vi "Configure Marker Search.vi"(7 "Marker Search (Max Peak)":T1, 8 "error in (no error)":errorcluster, 10 "Marker Number (1)":u32=1 min=1, 11 "SA-FSW in":refnum<class "SA-FSW.lvclass">) -> (0 "error out":errorcluster, 3 "SA-FSW out":refnum<class "SA-FSW.lvclass">)   [LabVIEW 2020, in "SA-FSW.lvclass"]
uses:
  SA-FSW.lvclass
  C:/Sandbox/RF Bench/Source Code/WiSpry Test Framework/Instruments/Instrument.lvclass
  Controls/Marker Search.ctl
  Instrument.lvclass/Instrument.ctl
  Instrument.lvclass
  Spectrum Analyzer.lvclass
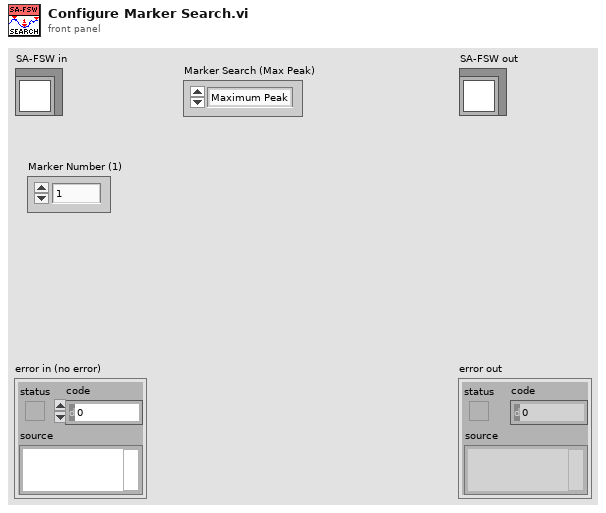
[diagram p1: front panel]
types:
  T1 = typedef "Spectrum Analyzer.lvclass/Marker Search.ctl" = enum16{"Maximum Peak", "Maximum Next", "Maximum Right", "Maximum Left", "Minimum Peak", "Minimum Next", "Minimum Right", "Minimum Left"}
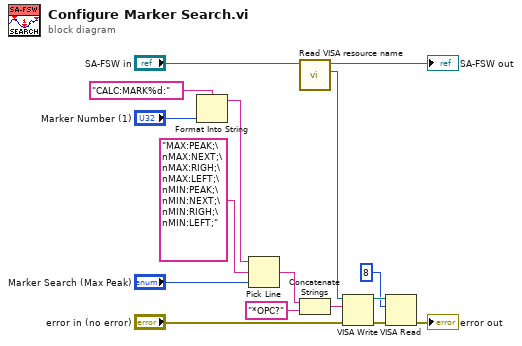
[diagram p0: block diagram]
diagram:
  n1 = Format Into String(format string="CALC:MARK%d:", "Marker Number (1)") -> (resulting string=w14:string)  [unwired: 2 in, 1 out]
  n2 = Pick Line(string ("")=w14, multi-line string="MAX:PEAK;\nMAX:NEXT;\nMAX:RIGH;\nMAX:LEFT;\nMIN:PEAK;\nMIN:NEXT;\nMIN:RIGH;\nMIN:LEFT;", line index="Marker Search (Max Peak)") -> (output string=w11:string)
  n3 = call "Read VISA resource name.vi"("Instrument in"="SA-FSW in") -> ("VISA resource name"=w6:refnum<visa-resource-name>, "Instrument out"=→"SA-FSW out":refnum<class "SA-FSW.lvclass">)  [unwired: 9 in]
  n4 = Concatenate Strings(w11, "*OPC?" ("string")) -> (w5:string)
  n5 = VISA Write(VISA resource name=w6, write buffer=w5, error in (no error)="error in (no error)") -> (VISA resource name out=w2:refnum<visa-resource-name>, error out=w3:errorcluster)  [unwired: 1 out]
  n6 = VISA Read(VISA resource name=w2, byte count=u32 8, error in (no error)=w3) -> (error out=→"error out":errorcluster)  [unwired: 3 out]
